vi "Call Vector Field Histogram.vi"(0 "LIDAR magn. (m)":dbl[](array[numeric]), 1 "max speed":dbl=0.7, 2 "Initialize?":bool, 5 "LIDAR angle (rad)":dbl[](array[numeric]), 7 "current heading (rad)":dbl, 9 "target heading (rad)":dbl, 11 "target distance":dbl, 12 "obstacle clearance (m)":dbl, 13 "thresholds":T1) -> (4 "command vx":dbl, 6 "command vy":dbl, 8 "command heading (rad)":dbl, 10 "histogram out":dbl[](array[numeric]), 15 "mask out":bool[](array[boolean]))   [LabVIEW 2018]
uses:
  <vilib>/Analysis/coordinate.llb/Angle Rotation (scalar).vi
  <vilib>/Analysis/coordinate.llb/Wrap Angle (scalar).vi
  <vilib>/Utility/AngleManip/Degrees to Radians (Scalar DBL).vi
  <vilib>/Utility/AngleManip/Radians to Degrees (Scalar DBL).vi
  <vilib>/robotics/Obstacle Avoidance/Advanced Vector Field Histogram/NI_Robotics_Vector Field Histogram.lvlib
  <vilib>/Utility/AngleManip/NI_AngleManipulation.lvlib
  <vilib>/Analysis/NI_AAL_Angle.lvlib
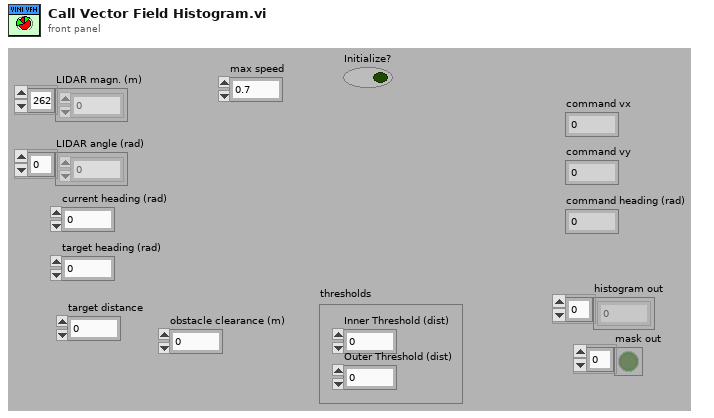
[diagram p1: front panel]
types:
  T1 = cluster{"Inner Threshold (dist)":dbl, "Outer Threshold (dist) ":dbl}
  T2 = cluster{"current heading (rad)":dbl, "target heading (rad)":dbl}
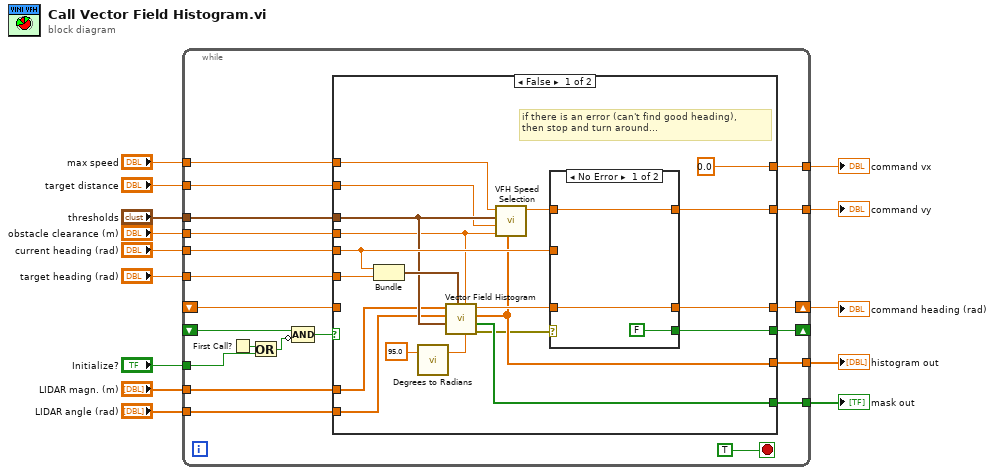
[diagram p0: block diagram]
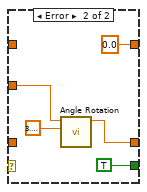
[diagram p2: hidden frame]
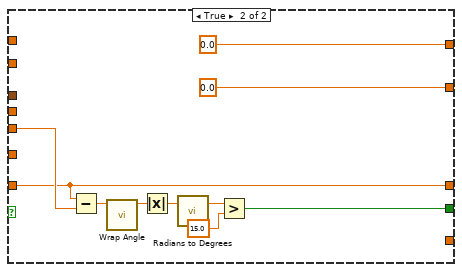
[diagram p3: hidden frame]
diagram:
  n1 = while {
    tunnel: [w34] -> w13
    tunnel: "max speed" -> [w33]
    tunnel: [w32] -> w11
    tunnel: "current heading (rad)" -> [w31]
    tunnel: [w30] -> w9
    shift-right: [w27] -> _
    shift-left: _ -> [w23]
    shift-right: [w26] -> w8
    shift-left: _ -> [w25]
    tunnel: [w35] -> w14
    tunnel: "thresholds" -> [w21]
    tunnel: "target distance" -> [w20]
    tunnel: "obstacle clearance (m)" -> [w19]
    tunnel: "target heading (rad)" -> [w18]
    tunnel: "LIDAR angle (rad)" -> [w17]
    tunnel: "LIDAR magn. (m)" -> [w16]
    tunnel: "Initialize?" -> [w15]
    stop <- TRUE stop-if-true
    n2 = First Call?() -> (First Call?: T/F=w28:bool)
    n3 = Or(x=w28, y=w15) -> (x .or. y?=w24:bool)
    n4 = Compound Arithmetic op=AND(w23, invert w24) -> (w22:bool)
    n5 = case shown="False" w22 {
      tunnel: [w55 0.0 ("VX")] -> w35
      tunnel: [0.0 0.0] -> w34
      tunnel: w33 -> [w52 _]
      tunnel: [w47 _] -> w32
      tunnel: w31 -> [w48 w71]
      tunnel: [w53 _] -> w30
      tunnel: [w46 w69] -> w27
      tunnel: [w50 w68] -> w26
      tunnel: w25 -> [_ w68]
      tunnel: w21 -> [w41 _]
      tunnel: w20 -> [w40 _]
      tunnel: w19 -> [w39 _]
      tunnel: w18 -> [w38 _]
      tunnel: w17 -> [w37 _]
      tunnel: w16 -> [w36 _]
      frame False {
        # "if there is an error (can't find good heading),\nthen stop and turn around..."
        n6 = Bundle("current heading (rad)"=w48, "target heading (rad)"=w38) -> (w44:T2)  [unwired: 1 in]
        n7 = call-poly <vilib>:"Degrees to Radians.vi"("angle (deg)"=95.0) -> ("angle (rad)"=w42:dbl)  [unwired: 2 in]
        n8 = call <vilib>:"Vector Field Histogram.vi"("maximum heading change (rad)"=w42, "obstacle clearance distance"=w39, "heading"=w44, "thresholds"=w41, "direction angles (rad)"=w37, "distances"=w36) -> ("error out"=w45:errorcluster, "mask"=w53:bool[], "histogram"=w47:dbl[], "chosen heading (rad)"=w51:dbl)  [unwired: 2 in]
        n9 = call "VFH Speed Selection.vi"("Histogram"=w47, "Obstacle Clearance"=w39, "Target Distance"=w40, "Thresholds"=w41, "Max Speed"=w52) -> ("Speed"=w49:dbl)  [unwired: 6 in]
        n10 = case shown="No Error" w45 {
          tunnel: [w57 0.0 ("VX")] -> w55
          tunnel: w51 -> [w58 _]
          tunnel: [w58 w59] -> w50
          tunnel: w49 -> [w57 _]
          tunnel: w48 -> [_ w61]
          tunnel: [FALSE TRUE] -> w46
          frame No Error {
          }
          frame Error {
            n11 = call-poly <vilib>:"Angle Rotation.vi"("counterclockwise rotation"=3.141592653589793, "angle"=w61) -> ("rotated angle"=w59:dbl)  [unwired: 8 in, 1 out]
          }
        }
      }
      frame True {
        n12 = Subtract(x=w68, y=w71) -> (x-y=w65:dbl)
        n13 = call-poly <vilib>:"Wrap Angle.vi"("angle in"=w65) -> ("angle out"=w64:dbl)  [unwired: 9 in, 1 out]
        n14 = Absolute Value(x=w64) -> (abs(x)=w67:dbl)
        n15 = call-poly <vilib>:"Radians to Degrees.vi"("angle (rad)"=w67) -> ("angle (deg)"=w66:dbl)  [unwired: 2 in]
        n16 = Greater?(x=w66, y=15.0) -> (0:w69:bool)
      }
    }
  }
  "command vy" <- w14
  "command vx" <- w13
  "histogram out" <- w11
  "mask out" <- w9
  "command heading (rad)" <- w8
